vi "sid_main.vi"(6 "idVar":cluster{"data":fxp<+/-,25,2>, "inputValid":bool}, 7 "sid.allowExternalRecord":bool, 8 "inputValid":bool, 9 "sid.p.params":T2={"sysIdOutputRate"=100, "sysIdWaveSize"=4092, "sysIdRepetitions"=50, "lowValue"=0.0, "highValue"=0.010009765625} {"sysIdOutputRate" min=10}, 10 "sid.p.start":bool, 11 "sid.i.height":fxp<+/-,31,4>) -> (0 "outputValid":bool, 1 "sid.running":bool, 2 "sid.o.height":fxp<+/-,43,16>, 3 "sid.o.count":u16, 4 "sid.s.recordPair":T1)   [LabVIEW 2016]
uses:
  <vilib>/rvi/Emulation/niFpgaEmulationIsFPGAContextNoSignature.vi
  <vilib>/rvi/Emulation/niFpgaSctlEmulationGetInTimedLoop.vi
  <vilib>/rvi/errors/niFpgaSetErrorForExecOnDevCompSimple.vi
  <vilib>/rvi/eio/common/nirviEmuReportErrorAndStop.vi
  <vilib>/rvi/DataTransferAndStorage/Container/Common/niFpgaContainerGetUniqueNameForEmu.vi
  <vilib>/rvi/FIFO/Fifo_Resource/nirvififoEmulationSetSize.vi
  <vilib>/rvi/FIFO/Fifo_Resource/nirviFifoEmulationQueueMgr.vi
  <instcachedir>/0/nirviFifoEmulationQueueMgr_E5CAEC123FF24DC58D834DCA3CDAA9B5.lvgen/nirviFifoEmulationQueueMgr_E5CAEC123FF24DC58D834DCA3CDAA9B5_009.vi
  <vilib>/Utility/error.llb/Clear Errors.vi
  <vilib>/rvi/FIFO/Fifo_Resource/nirvififoEmulationCreateLock.vi
  <vilib>/rvi/Emulation/niFpgaProcessEmulError.vi
  <vilib>/rvi/FIFO/Fifo_Resource/nirvififoEmulationObtainLock.vi
  <vilib>/rvi/FIFO/Fifo_Resource/nirvififoEmulationReleaseLock.vi
  <vilib>/rvi/occurrence/nirviWaitOnOccurrenceBase.vi
  <vilib>/rvi/errors/nirviReportUnexpectedCaseInternalError.vi
  <vilib>/rvi/errors/nirviReportUnexpectedCaseInternalError (U32).vi
  <instcachedir>/0/nirviFifoEmulationQueueMgr_E5CAEC123FF24DC58D834DCA3CDAA9B5.lvgen/nirviFifoEmulationQueueMgr_E5CAEC123FF24DC58D834DCA3CDAA9B5_003.vi
  <vilib>/rvi/FIFO/Fifo_Resource/nirvififoEmulationDetermineInputValidOut.vi
  <vilib>/rvi/DataTransferAndStorage/Container/XNode/niFpgaContainer.xnode
  <vilib>/rvi/FIFO/Fifo_Resource/nirvififoEmulationRead.vi
  <vilib>/rvi/FXPMathLib/FxpInterpret/XNode/nifxpmath_Interpret.xnode
  <vilib>/rvi/FIFO/Fifo_Resource/nirvififoEmulationWrite.vi
  <vilib>/rvi/interface/RandomDataEmulation/nirviRandomDataFpgaReadWriteTemplate.vi
  <vilib>/eio/EIONode/EIONode.xnode
  <instrlib>/_niInstr/Basic Elements/v1/FPGA/niInstr Basic Elements v1 FPGA.lvlib
  <vilib>/rvi/eio/common/nirviEmuTemplateMethod_errors.vi
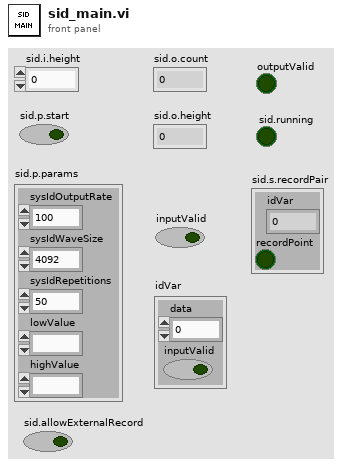
[diagram p1: front panel]
types:
  T1 = cluster{"idVar":fxp<+/-,25,2>, "recordPoint":bool}
  T2 = cluster{"sysIdOutputRate":u16, "sysIdWaveSize":u16, "sysIdRepetitions":u16, "lowValue":fxp<+/-,16,1>, "highValue":fxp<+/-,16,1>}
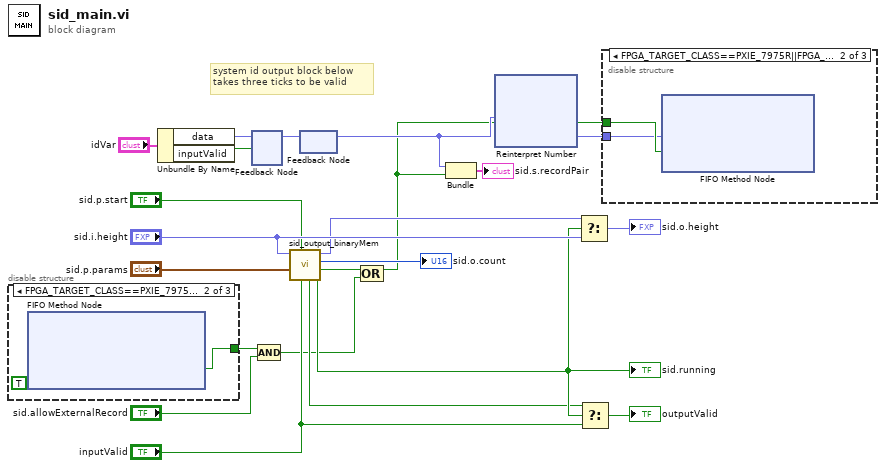
[diagram p0: block diagram]
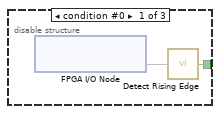
[diagram p2: hidden frame]
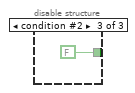
[diagram p3: hidden frame]
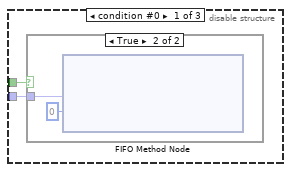
[diagram p4: hidden frame]
diagram:
  # "system id output block below \ntakes three ticks to be valid"
  n1 = disable-structure shown="FPGA_TARGET_CLASS==PXIE_7975R" {
    disable-tunnel: [w24 w26 FALSE ("edge detected")] -> w3
    frame condition #0 {
      n2 = xnode "FPGA I/O Node"() -> ("itc.sidRecord"=w23)  [unwired: 1 in, 1 out]
      n3 = call <instrlib>:"Detect Rising Edge.vi"("signal"=w23) -> ("edge detected"=w24:bool)  [unwired: 14 in]
    }
    frame condition #1 (active) {
      n4 = xnode ("FIFO Method Node")("Ready for Output"=TRUE) -> ("Output Valid"=w26:bool)  [unwired: 1 in, 2 out]
    }
    frame condition #2 {
    }
  }
  n5 = Unbundle By Name("idVar") -> ("data"=w6:fxp<+/-,25,2>, "inputValid"=w5:bool)
  n6 = feedback #1() -> (w7:fxp<+/-,25,2>)  [unwired: 1 in]
  n7 = feedback-in #1(w6, w5) -> ()
  n8 = Compound Arithmetic op=AND(w3, "sid.allowExternalRecord") -> (w2:bool)
  n9 = call "sid_output_binaryMem.vi"("inputValid"="inputValid", "startId"="sid.p.start", "sysIdParams"="sid.p.params", "feedbackHeight"="sid.i.height") -> ("sysIdRunning"=w16:bool, "recordPoint"=w12:bool, "sysIdRep"=→"sid.o.count":u16, "sid.o.height"=w19:fxp<+/-,28,1>, "outputValid"=w15:bool)  [unwired: 2 in, 1 out]
  "sid.running" <- w16
  n10 = feedback-in #2(w7) -> ()
  n11 = feedback #2() -> (w10:fxp<+/-,25,2>)  [unwired: 1 in]
  n12 = Compound Arithmetic op=OR(w12, w2) -> (w4:bool)
  n13 = Bundle("data"=w10, w4) -> (→"sid.s.recordPair":cluster{"data":fxp<+/-,25,2>, bool})  [unwired: 1 in]
  n14 = xnode "Reinterpret Number"("x"=w10) -> ("y"=w9:fxp<+/-,25,17>)
  n15 = Select(t=w19, s=w16, f="sid.i.height") -> (s? t:f=→"sid.o.height":fxp<+/-,31,4>)
  n16 = Select(t=w15, s=w16, f="inputValid") -> (s? t:f=→"outputValid":bool)
  n17 = disable-structure shown="FPGA_TARGET_CLASS==PXIE_7975R||FPGA_TARGET_CLASS==PXI_7954R" {
    disable-tunnel: w9 -> [w29 w32 _]
    disable-tunnel: w4 -> [w28 w33 _]
    frame condition #0 {
      n18 = case shown="True" w28 {
        tunnel: w29 -> [_ w30]
        frame False {
        }
        frame True {
          n19 = xnode ("FIFO Method Node")("Element"=w30, "Timeout"=0) -> ()  [unwired: 1 in, 2 out]
        }
      }
    }
    frame condition #1 (active) {
      n20 = xnode ("FIFO Method Node")("Element"=w32, "Input Valid"=w33) -> ()  [unwired: 1 in, 2 out]
    }
    frame condition #2 {
    }
  }
